vi "foorloop.vi"() -> ()   [LabVIEW 2020]
panel:
  out "number (0 to 1)":dbl
  out "Numeric 2":i32
  in  "Numeric":i32
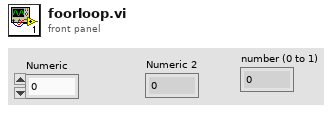
[diagram p1: front panel]
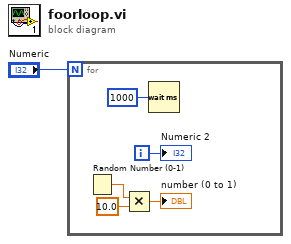
[diagram p0: block diagram]
diagram:
  n1 = for {
    N: "Numeric" -> [_]
    i -> [w6]
    n2 = Random Number (0-1)() -> (number: 0 to 1=w4:dbl)
    n3 = Multiply(x=w4, y=10.0) -> (x*y=→"number (0 to 1)":dbl)
    n4 = Wait (ms)(milliseconds to wait=u32 1000) -> ()  [unwired: 1 out]
    "Numeric 2" <- w6
  }
